vi "AlliGator Compute INT - G2 Images.vi"(4 "INT Images":T1[](array[typedef]), 6 "Sum(INT)":T1, 7 "G2 Images":T1[](array[typedef]), 8 "error in":errorcluster, 9 "Min(G2)":T1, 10 "Max(G2)":T1, 11 "Sum(G2)":T1) -> (0 "error out":errorcluster, 1 "Min(INT - G2)":T1, 2 "Max(INT - G2)":T1, 3 "Sum(INT - G2)":T1, 5 "INT - G2":T1[](array[typedef]))   [LabVIEW 2021, in "AlliGator Dual-Channel Datasets.lvlib"]
doc: "Computes INT - G2."
uses:
  AlliGator Dual-Channel Datasets.lvlib
  <vilib>/vision/Image Controls.llb/IMAQ Image.ctl
  <vilib>/vision/NI_Vision_Development_Module.lvlib
  Image/Image.lvlib
  Utilities/Utilities.lvlib
panel:
  # "see the AlliGator License on the block diagram (Ctrl+E or Window:Show Block Diagram)"
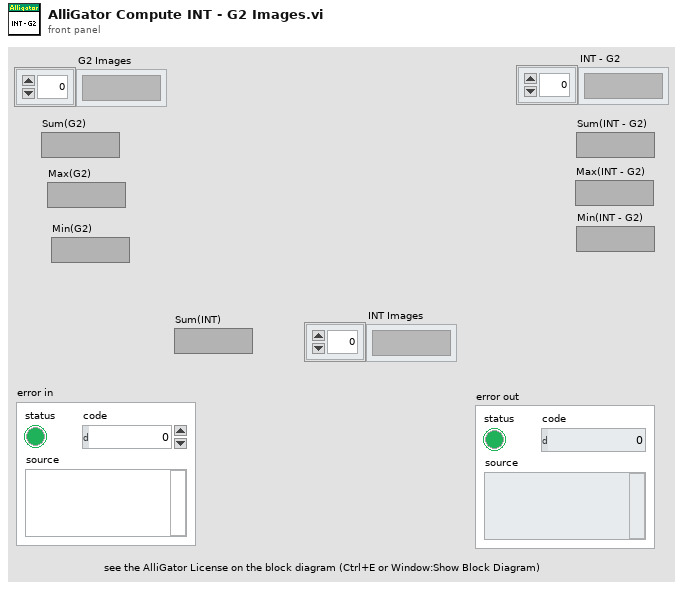
[diagram p1: front panel]
types:
  T1 = typedef "IMAQ Image.ctl" = refnum<image>
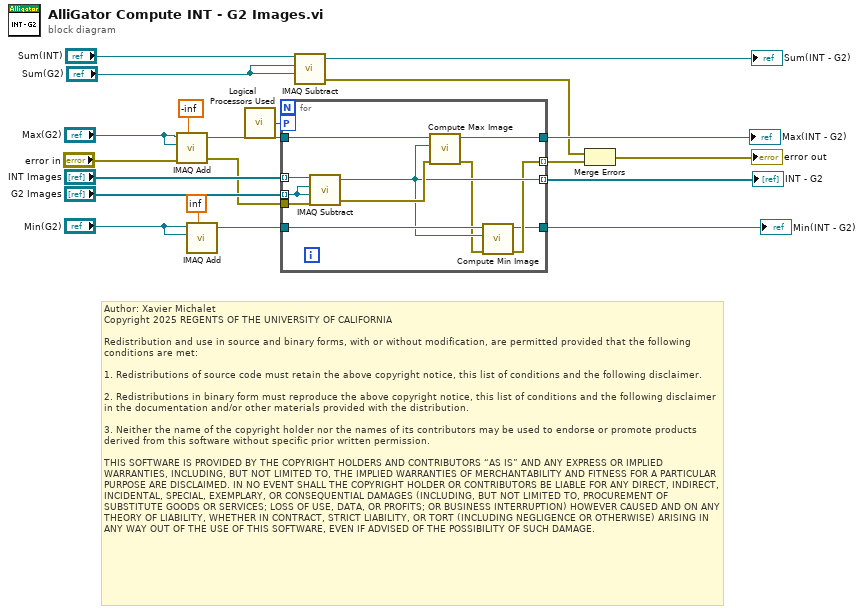
[diagram p0: block diagram]
diagram:
  # "Author: Xavier Michalet\nCopyright 2025 REGENTS OF THE UNIVERSITY OF CALIFORNIA\n\nRedistribution and use in source and binary forms, with or without modification, are permitted provided that the following conditions are met:\n\n1. Redistributions of source code must retain the above copyright notice, this list of conditions and the following disclaimer.\n\n2. Redistributions in binary form must reproduce the above copyright notice, this list of conditions and the following disclaimer in the documentation and/or other materials provided with the distribution.\n\n3. Neither the name of the copyright holder nor the names of its contributors may be used to endorse or promote products derived from this software without specific prior written permission.\n\nTHIS SOFTWARE IS PROVIDED BY THE COPYRIGHT HOLDERS AND CONTRIBUTORS “AS IS” AND ANY EXPRESS OR IMPLIED WARRANTIES, INCLUDING, BUT NOT LIMITED TO, THE IMPLIED WARRANTIES OF MERCHANTABILITY AND FITNESS FOR A PARTICULAR PURPOSE ARE DISCLAIMED. IN NO EVENT SHALL THE COPYRIGHT HOLDER OR CONTRIBUTORS BE LIABLE FOR ANY DIRECT, INDIRECT, INCIDENTAL, SPECIAL, EXEMPLARY, OR CONSEQUENTIAL DAMAGES (INCLUDING, BUT NOT LIMITED TO, PROCUREMENT OF SUBSTITUTE GOODS OR SERVICES; LOSS OF USE, DATA, OR PROFITS; OR BUSINESS INTERRUPTION) HOWEVER CAUSED AND ON ANY THEORY OF LIABILITY, WHETHER IN CONTRACT, STRICT LIABILITY, OR TORT (INCLUDING NEGLIGENCE OR OTHERWISE) ARISING IN ANY WAY OUT OF THE USE OF THIS SOFTWARE, EVEN IF ADVISED OF THE POSSIBILITY OF SUCH DAMAGE."
  n1 = call "IMAQ Add"("Image Src A"="Max(G2)", "Constant"=-inf, "Image Dst"="Max(G2)", "error in (no error)"="error in") -> ("Image Dst Out"=w5:T1, "error out"=w7:errorcluster)  [unwired: 3 in]
  n2 = call "IMAQ Add"("Image Src A"="Min(G2)", "Constant"=inf, "Image Dst"="Min(G2)") -> ("Image Dst Out"=w1:T1)  [unwired: 4 in, 1 out]
  n3 = call "Logical Processors Used.vi"() -> ("# Logical Processor Used"=w3:i32)  [unwired: 6 in]
  n4 = for {
    tunnel: "INT Images" -> [w31] mode=indexing
    tunnel: "G2 Images" -> [w30] mode=indexing
    workers-P: w3 -> [_]
    tunnel: [w24] -> w14 mode=indexing
    tunnel: w5 -> [w29]
    tunnel: [w22] -> w6 mode=indexing
    tunnel: w7 -> [w27]
    tunnel: [w26] -> w18
    tunnel: w1 -> [w25]
    tunnel: [w21] -> w9
    n5 = call "IMAQ Subtract"("Image Src A"=w31, "Image Dst"=w30, "Image Src B"=w30, "error in (no error)"=w27) -> ("Image Dst Out"=w24:T1, "error out"=w28:errorcluster)  [unwired: 3 in]
    n6 = call "Compute Max Image.vi"("error in (no error)"=w28, "New Image"=w24, "Max Image Dst"=w29) -> ("error out"=w23:errorcluster, "Max Image"=w26:T1)  [unwired: 7 in]
    n7 = call "Compute Min Image.vi"("error in (no error)"=w23, "New Image"=w24, "Min Image Dst"=w25) -> ("error out"=w22:errorcluster, "Min Image"=w21:T1)  [unwired: 7 in]
  }
  "Max(INT - G2)" <- w18
  "INT - G2" <- w14
  "Min(INT - G2)" <- w9
  n8 = call "IMAQ Subtract"("Image Src A"="Sum(INT)", "Image Dst"="Sum(G2)", "Image Src B"="Sum(G2)") -> ("Image Dst Out"=→"Sum(INT - G2)":T1, "error out"=w8:errorcluster)  [unwired: 4 in]
  n9 = Merge Errors(w8, w6) -> (→"error out":errorcluster)
